vi "UI - Initiate Connection v2.vi"(8 "error in (no error)":errorcluster, 10 "Controller Address":string, 11 "Message Queue":refnum<queue>) -> (0 "error out":errorcluster, 1 "Connected?":bool)   [LabVIEW 2017]
uses:
  Message Queue/Message Cluster.ctl
  controls/Variable References.ctl
  controls/Control State.ctl
  Globals/Global - Configuration Options.vi
  Globals/Global - UI Stream and Variable Connections.vi
  Message Queue/Message Queue.lvlib
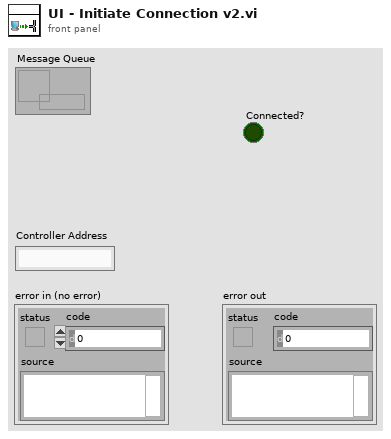
[diagram p1: front panel]
types:
  T1 = typedef "Message Queue.lvlib/Message Cluster.ctl" = cluster{"Message":string, "Message Data":variant}
  T2 = typedef "Variable References.ctl" = cluster{"CPU Usage":refnum<k21>, "Contiguous Memory":refnum<k21>, "Control Mode":refnum<k21>, "Control Loop Period":refnum<k21>, "Input Values":refnum<k21>, "Output Values":refnum<k21>}
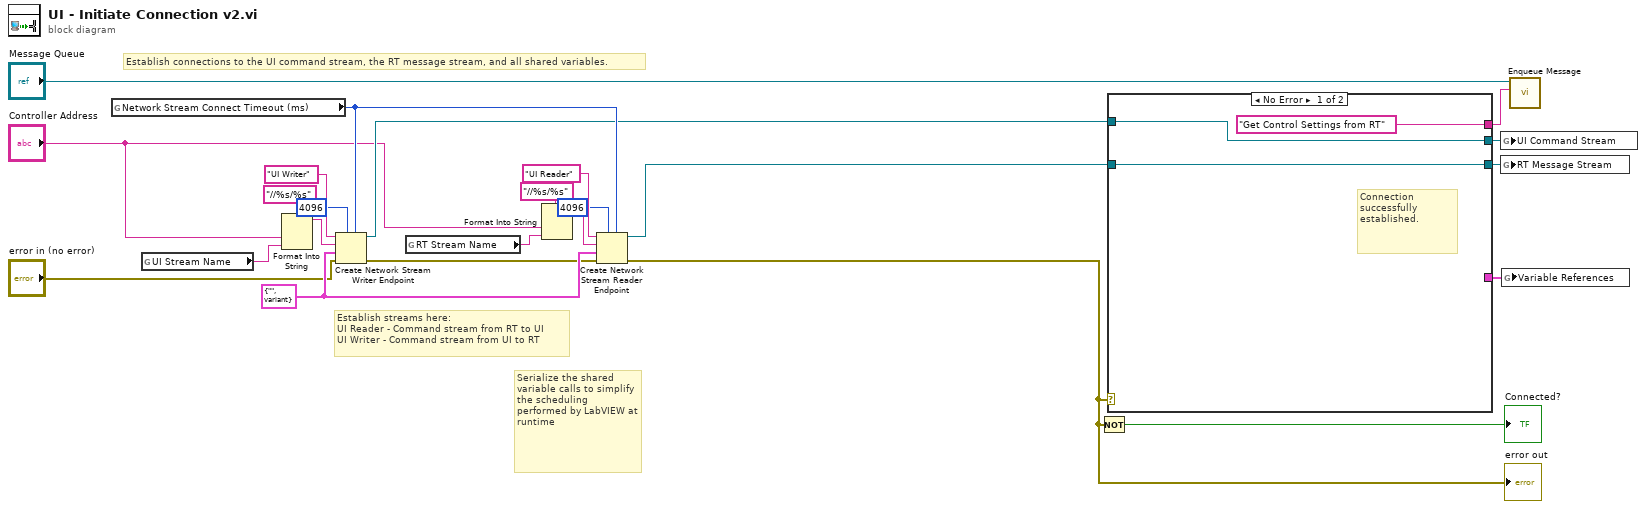
[diagram p0: block diagram]
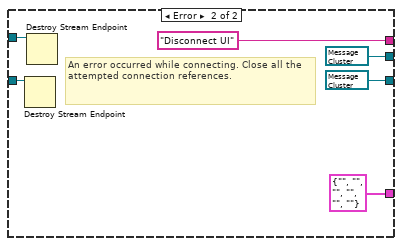
[diagram p2: hidden frame]
diagram:
  w15 = T1 {"Message"="", "Message Data"=variant} ("Message Cluster")
  # "Establish connections to the UI command stream, the RT message stream, and all shared variables."
  # "Establish streams here:\nUI Reader - Command stream from RT to UI\nUI Writer - Command stream from UI to RT"
  # "Serialize the shared variable calls to simplify the scheduling performed by LabVIEW at runtime"
  n1 = global read "Global - Configuration Options.vi" "Network Stream Connect Timeout (ms)"() -> (w14:i32)
  n2 = global read "Global - Configuration Options.vi" "UI Stream Name"() -> (w22:string)
  n3 = Format Into String(format string="//%s/%s", "Controller Address", w22) -> (resulting string=w21:string)  [unwired: 2 in, 1 out]
  n4 = Create Network Stream Writer Endpoint(5:w14, 7:4096 ("writer buffer size"), 8:"error in (no error)", 9:w15, 10:w21, 11:"UI Writer" ("writer name")) -> (0:w5:errorcluster, 3:w13:refnum<k21>)  [unwired: 1 in]
  n5 = global read "Global - Configuration Options.vi" "RT Stream Name"() -> (w19:string)
  n6 = Format Into String(format string="//%s/%s", "Controller Address", w19) -> (resulting string=w18:string)  [unwired: 2 in, 1 out]
  n7 = Create Network Stream Reader Endpoint(5:w14, 7:4096 ("reader buffer size"), 8:w5, 9:w15, 10:w18, 11:"UI Reader" ("reader name")) -> (0:w1:errorcluster, 3:w12:refnum<k21>)  [unwired: 1 in]
  "error out" <- w1
  n8 = Not(x=w1) -> (.not. x?=→"Connected?":bool)
  n9 = case shown="No Error" w1 {
    tunnel: w13 -> [w25 w32]
    tunnel: w12 -> [w27 w33]
    tunnel: [_ T2 {"CPU Usage"="", "Contiguous Memory"="", "Control Mode"="", "Control Loop Period"="", "Input Values"="", "Output Values"=""} ("Variable References")] -> w11
    tunnel: [w27 refnum<k21> refnum] -> w10
    tunnel: [w25 refnum<k21> refnum] -> w9
    tunnel: ["Get Control Settings from RT" "Disconnect UI"] -> w7
    frame No Error {
      # "Connection successfully established."
    }
    frame Error {
      # "An error occurred while connecting. Close all the attempted connection references."
      n10 = Destroy Stream Endpoint(11:w33) -> ()  [unwired: 1 in, 1 out]
      n11 = Destroy Stream Endpoint(11:w32) -> ()  [unwired: 1 in, 1 out]
    }
  }
  n12 = global write "Global - UI Stream and Variable Connections.vi" "UI Command Stream"(w9) -> ()
  n13 = global write "Global - UI Stream and Variable Connections.vi" "RT Message Stream"(w10) -> ()
  n14 = global write "Global - UI Stream and Variable Connections.vi" "Variable References"(w11) -> ()
  n15 = call "Enqueue Message.vi"("Message"=w7, "Message Queue"="Message Queue") -> ()  [unwired: 8 in, 2 out]
